vi "9224_Initialize.vi"(7 "Module Model":T1, 8 "error in (no error)":errorcluster, 9 "Slot Settings":T2, 11 "9224 in":refnum<class "9224.lvclass">) -> (0 "error out":errorcluster, 3 "9224 out":refnum<class "9224.lvclass">)   [LabVIEW 2020, in "Modules.lvlib" / "9224.lvclass"]
uses:
  9224.lvclass
  C:/Users/nitest/Desktop/Git 2020/niveristand-scan-engine-module-libraries/Source/RSI Module/RSI Module.lvclass
  RSI Module/Slot Settings.ctl
  RSI Module/Module Models.ctl
  RSI Module/Channels.ctl
  RSI Module/Channel Type.ctl
  Conversion Time.ctl
  9224.lvclass/9224.ctl
  RSI Module/RSI Module.lvclass
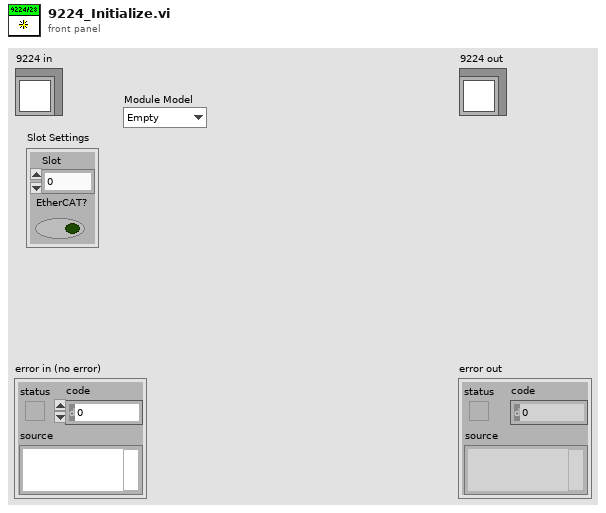
[diagram p1: front panel]
types:
  T1 = typedef "Modules.lvlib/RSI Module.lvclass/Module Models.ctl" = enum16{"Empty", "NI 9201", "NI 9203", "NI 9205", "NI 9206", "NI 9207", "NI 9208", "NI 9209", "NI 9210", "NI 9211", "NI 9212", "NI 9213", "NI 9214", "NI 9215", "NI 9216", "NI 9217", "NI 9219", "NI 9220", "NI 9221", "NI 9222", "NI 9223", "NI 9224", "NI 9225", "NI 9226", "NI 9227", "NI 9228", "NI 9229", "NI 9233", "NI 9234", "NI 9235", "NI 9236", "NI 9237", "NI 9239", "NI 9242", "NI 9244", "NI 9253", "NI 9263", "NI 9264", "NI 9265", "NI 9266", "NI 9269", "NI 9344", "NI 9350", "NI 9375", "NI 9401", "NI 9402", "NI 9403", "NI 9411", "NI 9421", "NI 9422", "NI 9423", "NI 9425", "NI 9426", "NI 9435", "NI 9436", "NI 9437", "NI 9472", "NI 9474", "NI 9475", "NI 9476", "NI 9477", "NI 9478", "NI 9481", "NI 9482", "NI 9485"}
  T2 = typedef "Modules.lvlib/RSI Module.lvclass/Slot Settings.ctl" = cluster{"Slot":u32, "EtherCAT?":bool}
  T3 = typedef "Modules.lvlib/RSI Module.lvclass/Channels.ctl" = cluster{"# Input Channels":i32, "# Output Channels":i32, "Channel Type":T4, "Units":string}
  T4 = typedef "Modules.lvlib/RSI Module.lvclass/Channel Type.ctl" = enum16{"Analog", "Digital"}
  T5 = typedef "Modules.lvlib/9224.lvclass/Conversion Time.ctl" = u16
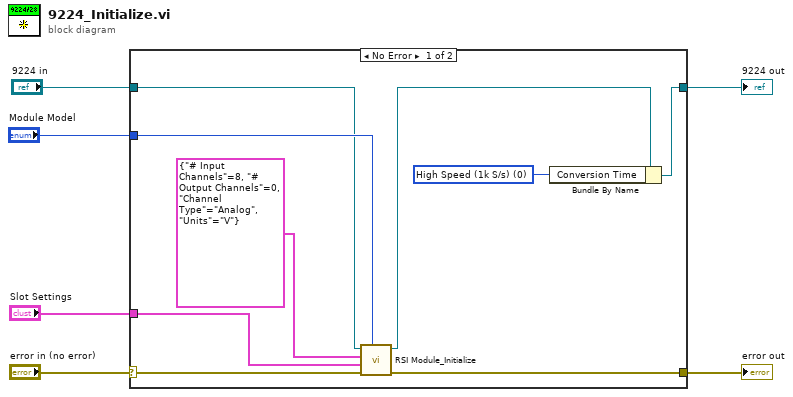
[diagram p0: block diagram]
diagram:
  n1 = case shown="No Error" "error in (no error)" {
    selector: "error in (no error)" -> [w15 w16]
    tunnel: [w9 w16] -> w3
    tunnel: [w11 w17] -> w4
    tunnel: "9224 in" -> [w12 w17]
    tunnel: "Slot Settings" -> [w14 _]
    tunnel: "Module Model" -> [w13 _]
    frame No Error {
      w8 = T5 0 items=["High Speed (1k S/s)", "Medium Speed (100 S/s)", "Medium Resolution (50/60Hz Rejection - 12 S/s)", "High Resolution (50/60Hz rejection - 2 S/s)"] ("Conversion Time")
      n2 = call "RSI Module_Initialize.vi"("Module Model"=w13, "error in (no error)"=w15, "Slot Settings"=w14, "Channels"=T3 {"# Input Channels"=8, "# Output Channels"=0, "Channel Type"=enum."Analog", "Units"="V"}, "RSI Module in"=w12) -> ("error out"=w9:errorcluster, "RSI Module out"=w7:refnum<class "9224.lvclass">)  [unwired: 5 in]
      n3 = Bundle By Name(cluster=w7, "Conversion Time"=w8) -> (w11:refnum<class "9224.lvclass">)
    }
    frame Error {
    }
  }
  "error out" <- w3
  "9224 out" <- w4
